vi "Set Calibrator Range.vi"(8 "error in (no error)":errorcluster, 10 "Calibrator Range (0: 10 mV)":u32(ring) items=["10 mV", "25 mV", "100 mV", "250 mV", "1 V", "2.5 V", "Res 50 ohm", "Res 1 Mohm", "Capacitance", "DC", "AC"], 11 "VISA resource name":refnum<visa-resource-name>) -> (0 "error out":errorcluster, 3 "VISA resource name out":refnum<visa-resource-name>)   [LabVIEW 2014, in "Fluke 5XXX Series Multicalibrators.lvlib"]
doc: "This VI programs the instrument range in Pulse, Impedance & Capacitance Measurement and Overload scope modes.\n\nNote:\n\nThis VI is available only for instrument models 5500A and 5520A with oscilloscope option SC600 (SC1100)."
uses:
  Fluke 5XXX Series Multicalibrators.lvlib
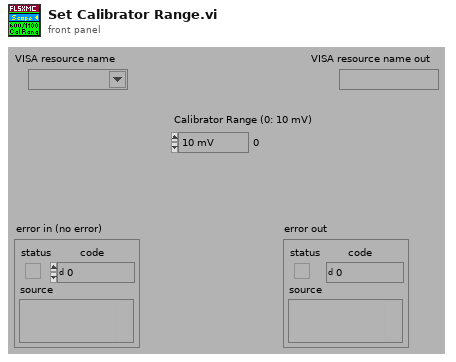
[diagram p1: front panel]
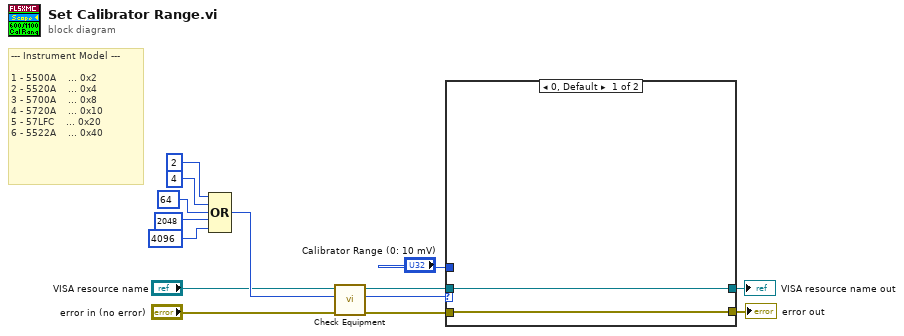
[diagram p0: block diagram]
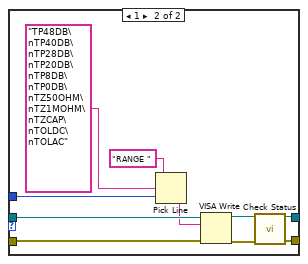
[diagram p2: hidden frame]
diagram:
  # "--- Instrument Model ---\n\n1 - 5500A    ... 0x2\n2 - 5520A    ... 0x4\n3 - 5700A    ... 0x8\n4 - 5720A    ... 0x10\n5 - 57LFC    ... 0x20\n6 - 5522A    ... 0x40"
  n1 = Compound Arithmetic op=OR(2 ("Numeric"), 4 ("Numeric"), 64 ("Numeric"), 2048 ("Numeric"), 4096 ("Numeric")) -> (w9:i32)
  n2 = call "Check Equipment.vi"("error in (no error)"="error in (no error)", "Bit Mask"=w9, "VISA resource name"="VISA resource name") -> ("error out"=w12:errorcluster, "Present?"=w11:u32, "VISA resource name out"=w10:refnum<visa-resource-name>)  [unwired: 6 in]
  n3 = case shown="0, Default" w11 {
    tunnel: [w15 w23] -> w3
    tunnel: w12 -> [w16 w21]
    tunnel: w10 -> [w15 w22]
    tunnel: [w16 w26] -> w4
    tunnel: "Calibrator Range (0: 10 mV)" -> [_ w19]
    frame 0, Default {
    }
    frame 1 {
      n4 = Pick Line(string ("")="RANGE " ("Reset Command"), multi-line string="TP48DB\nTP40DB\nTP28DB\nTP20DB\nTP8DB\nTP0DB\nTZ50OHM\nTZ1MOHM\nTZCAP\nTOLDC\nTOLAC", line index=w19) -> (output string=w18:string)
      n5 = VISA Write(VISA resource name=w22, write buffer=w18, error in (no error)=w21) -> (VISA resource name out=w24:refnum<visa-resource-name>, error out=w25:errorcluster)  [unwired: 1 out]
      n6 = call "Check Status.vi"("VISA resource name"=w24, "error in (no error)"=w25) -> ("VISA resource name out"=w23:refnum<visa-resource-name>, "error out"=w26:errorcluster)  [unwired: 12 in]
    }
  }
  "VISA resource name out" <- w3
  "error out" <- w4
